vi "Load Config.vi"(8 "error in (no error)":errorcluster, 11 "DAQmxThermocoupleChannel in":refnum<class "TCChannel.lvclass">) -> (0 "error out":errorcluster, 3 "DAQmxThermocoupleChannel out":refnum<class "TCChannel.lvclass">)   [LabVIEW 2020, in "VolatusDAQConfig.lvlib" / "TCChannel.lvclass"]
uses:
  TCChannel.lvclass
  C:/dev/lv20CE/relink/lv-volatus/VolatusConfig/VolatusConfigElement/VolatusConfigElement.lvclass
  Temperature Units.ctl
  TC Type.ctl
  VolatusConfig/VolatusConfigElement/VolatusConfigElement.lvclass/VolatusConfigElement.ctl
  TCChannel.lvclass/TCChannel.ctl
  VolatusConfig/VolatusConfigElement/Element.vi
  VolatusConfig/VolatusConfigElement/VolatusConfigElement.lvclass
  lv-cdm/CDM-Config/Config Element/Config Element.lvclass
  VolatusDAQConfig.lvlib
  C:/dev/lv20CE/relink/lv-volatus/VolatusDAQConfig/DAQmxChannel/DAQmxChannel.lvclass
  C:/dev/lv20CE/relink/lv-volatus/VolatusConfig/Channel/Channel.lvclass
  C:/dev/lv20CE/relink/lv-volatus/VolatusDAQConfig/DAQmxThermocoupleChannel/TCChannel.lvclass
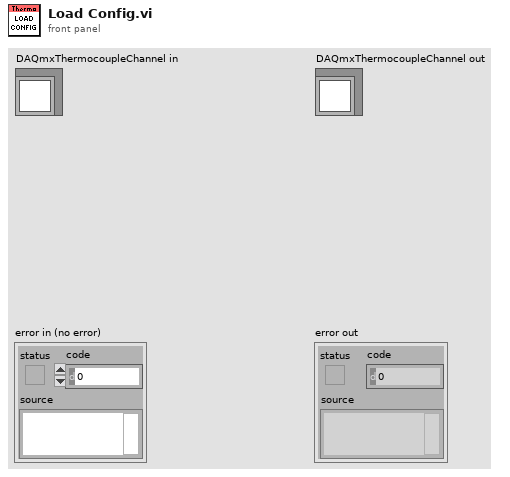
[diagram p1: front panel]
types:
  T1 = typedef "VolatusDAQConfig.lvlib/TC Type.ctl" = enum16{"J", "K", "N", "R", "S", "T", "B", "E"}
  T2 = typedef "VolatusDAQConfig.lvlib/Temperature Units.ctl" = enum16{"C", "F", "K", "R"}
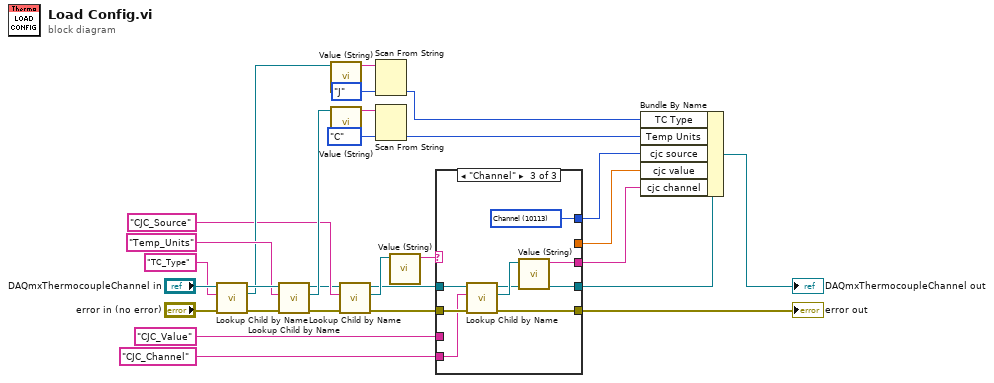
[diagram p0: block diagram]
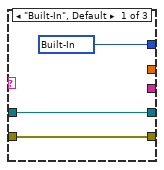
[diagram p2: hidden frame]
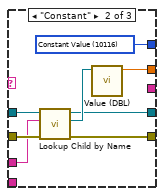
[diagram p3: hidden frame]
diagram:
  n1 = call "Lookup Child by Name.vi"("error in (no error)"="error in (no error)", "Child Name"="TC_Type", "VolatusConfigElement in"="DAQmxThermocoupleChannel in") -> ("error out"=w28:errorcluster, "Child"=w23:refnum<class "Config Element.lvclass">, "VolatusConfigElement out"=w25:refnum<class "TCChannel.lvclass">)  [unwired: 5 in, 1 out]
  n2 = call "Lookup Child by Name.vi"("error in (no error)"=w28, "Child Name"="Temp_Units", "VolatusConfigElement in"=w25) -> ("error out"=w13:errorcluster, "Child"=w22:refnum<class "Config Element.lvclass">, "VolatusConfigElement out"=w14:refnum<class "TCChannel.lvclass">)  [unwired: 5 in, 1 out]
  n3 = call "Value (String).vi"("Config Element in"=w23) -> ("String Value"=w19:string)  [unwired: 9 in, 1 out]
  n4 = call "Value (String).vi"("Config Element in"=w22) -> ("String Value"=w21:string)  [unwired: 9 in, 1 out]
  n5 = call "Lookup Child by Name.vi"("error in (no error)"=w13, "Child Name"="CJC_Source", "VolatusConfigElement in"=w14) -> ("error out"=w9:errorcluster, "Child"=w12:refnum<class "Config Element.lvclass">, "VolatusConfigElement out"=w10:refnum<class "TCChannel.lvclass">)  [unwired: 5 in, 1 out]
  n6 = Scan From String(input string=w19, default 1=TC_Type."J" ("TC Type")) -> (output 1=w16:T1)  [unwired: 3 in, 3 out]
  n7 = Scan From String(input string=w21, default 1=Temperature_Units."C" ("Temp Units")) -> (output 1=w17:T2)  [unwired: 3 in, 3 out]
  n8 = call "Value (String).vi"("Config Element in"=w12) -> ("String Value"=w11:string)  [unwired: 9 in, 1 out]
  n9 = case shown="\"Channel\"" w11 {
    tunnel: w10 -> [w31 w40 w48]
    tunnel: w9 -> [w30 w39 w47]
    tunnel: "CJC_Value" ("Child Name") -> [_ w38 _]
    tunnel: [w30 w36 w45] -> w7
    tunnel: [w31 w35 w44] -> w5
    tunnel: [w32 w34 w43] -> w6
    tunnel: [_ w33 _] -> w3
    tunnel: "CJC_Channel" ("Child Name") -> [_ _ w42]
    tunnel: [_ _ w41] -> w1
    frame "Built-In", Default {
      w32 = 10200 items=["Built-In"=10200, "Constant Value"=10116, "Channel"=10113] ("cjc source")
    }
    frame "Constant" {
      w34 = 10116 items=["Built-In"=10200, "Constant Value"=10116, "Channel"=10113] ("cjc source")
      n10 = call "Lookup Child by Name.vi"("error in (no error)"=w39, "Child Name"=w38, "VolatusConfigElement in"=w40) -> ("error out"=w36:errorcluster, "Child"=w37:refnum<class "Config Element.lvclass">, "VolatusConfigElement out"=w35:refnum<class "TCChannel.lvclass">)  [unwired: 5 in, 1 out]
      n11 = call "Value (DBL).vi"("Config Element in"=w37) -> ("DBL Value"=w33:dbl)  [unwired: 9 in, 1 out]
    }
    frame "Channel" {
      w43 = 10113 items=["Built-In"=10200, "Constant Value"=10116, "Channel"=10113] ("cjc source")
      n12 = call "Lookup Child by Name.vi"("error in (no error)"=w47, "Child Name"=w42, "VolatusConfigElement in"=w48) -> ("error out"=w45:errorcluster, "Child"=w46:refnum<class "Config Element.lvclass">, "VolatusConfigElement out"=w44:refnum<class "TCChannel.lvclass">)  [unwired: 5 in, 1 out]
      n13 = call "Value (String).vi"("Config Element in"=w46) -> ("String Value"=w41:string)  [unwired: 9 in, 1 out]
    }
  }
  "error out" <- w7
  n14 = Bundle By Name(cluster=w5, "TC Type"=w16, "Temp Units"=w17, "cjc source"=w6, "cjc value"=w3, "cjc channel"=w1) -> (→"DAQmxThermocoupleChannel out":refnum<class "TCChannel.lvclass">)
